vi "AB Update Dest Dir.vi"(8 "error in (no error)":errorcluster, 11 "Build in":refnum<class "AB_Build.lvclass">) -> (0 "error out":errorcluster, 3 "Build out":refnum<class "AB_Build.lvclass">)   [LabVIEW 2020]
uses:
  <vilib>/AppBuilder/AB_Classes/Build/AB_Build.lvclass
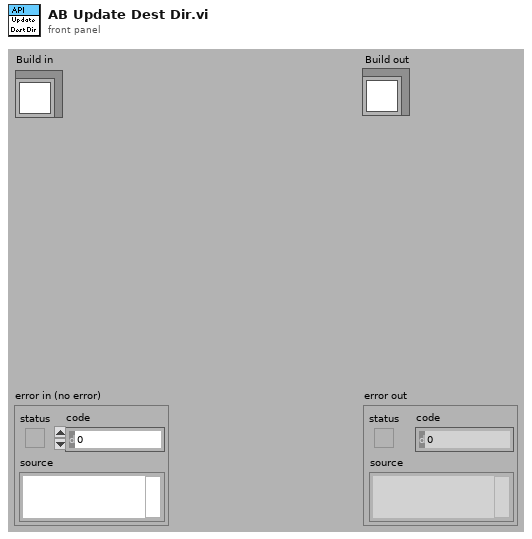
[diagram p1: front panel]
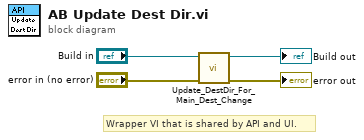
[diagram p0: block diagram]
diagram:
  # "Wrapper VI that is shared by API and UI."
  n1 = call-dynamic "Update_DestDir_For_Main_Dest_Change.vi"("error in (no error)"="error in (no error)", "AB_Build in"="Build in") -> ("error out"=→"error out":errorcluster, "AB_Build out"=→"Build out":refnum<class "AB_Build.lvclass">)  [unwired: 8 in]
